vi "Start Acquisition.vi"(8 "error in (no error)":errorcluster, 11 "session In":T2) -> (0 "error out":errorcluster, 3 "session out":T1)   [LabVIEW 2023]
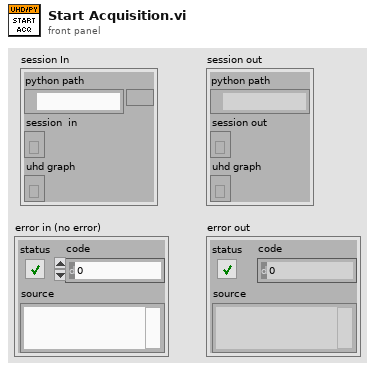
[diagram p1: front panel]
types:
  T1 = cluster{"python path":path, "session out ":refnum<k35>, "uhd graph":refnum<k38>}
  T2 = cluster{"python path":path, "session  in":refnum<k35>, "uhd graph":refnum<k38>}
  T3 = cluster{"python path":path, "session out":refnum<k35>, "uhd graph":refnum<k38>}
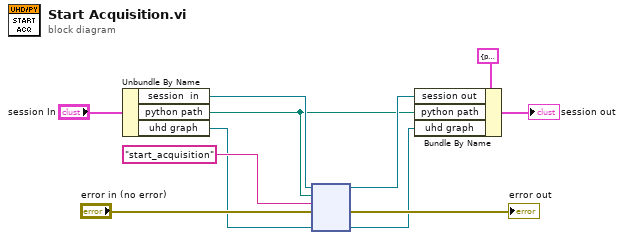
[diagram p0: block diagram]
diagram:
  n1 = Unbundle By Name("session In") -> ("session  in"=w5:refnum<k35>, "python path"=w1:path, "uhd graph"=w4:refnum<k38>)
  n2 = node(w5, w1, "start_acquisition" ("function name"), "error in (no error)", w4) -> (w2:refnum<k35>, →"error out":errorcluster, w3:refnum<k38>)  [unwired: 2 in, 2 out]
  n3 = Bundle By Name(cluster=T3 {"python path"=path "", "session out"=refnum, "uhd graph"=refnum}, "session out"=w2, "python path"=w1, "uhd graph"=w3) -> (→"session out":T3)
